vi "read_waveform_length.vi"(2 "N":u32, 3 "path":string) -> (1 "length":i32)   [LabVIEW 2022 SP3]
uses:
  <vilib>/Waveform/WDTFileIO.llb/Read Waveform from File.vi
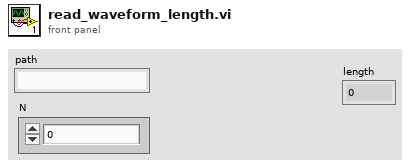
[diagram p1: front panel]
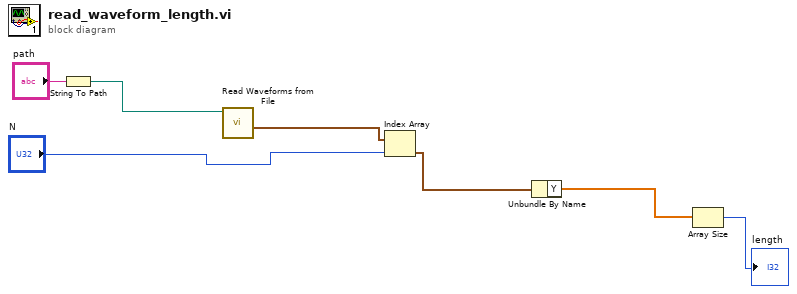
[diagram p0: block diagram]
diagram:
  n1 = String To Path(string="path") -> (path=w4:path)
  n2 = call-poly <vilib>:"Read Waveforms from File.vi"("file path (dialog if empty)"=w4) -> ("all waveforms in record"=w7:waveform(dbl)[])  [unwired: 5 in, 3 out]
  n3 = Index Array(array=w7, index="N") -> (element=w5:waveform(dbl))
  n4 = Unbundle By Name(w5) -> ("Y"=w2:dbl[])
  n5 = Array Size(array=w2) -> (size(s)=→"length":i32)
